vi "Get Section Name.vi"(11 "Section Name in":refnum<class "Section Name.lvclass">) -> (2 "Section Name":string, 3 "Section Name out":refnum<class "Section Name.lvclass">)   [LabVIEW 2019, in "Electronic Datasheet.lvlib" / "Section Name.lvclass"]
uses:
  Section Name.lvclass
  Section Name.lvclass/Section Name.ctl
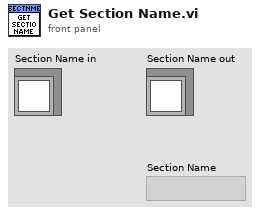
[diagram p1: front panel]
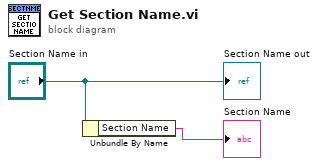
[diagram p0: block diagram]
diagram:
  n1 = Unbundle By Name("Section Name in") -> ("Section Name"=→"Section Name":string)
  "Section Name out" <- "Section Name in"
